vi "Create Tree.vi"(8 "Error In":errorcluster, 10 "Graves":T1[](array[typedef]), 11 "TreeControl In":refnum<vi>) -> (0 "Error Out":errorcluster, 3 "TreeControl Out":refnum<vi>)   [LabVIEW 2017, in "Graveyard.lvlib"]
uses:
  Graveyard.lvlib
  VI Bookmark.ctl
  VI Information.ctl
  Application Information.ctl
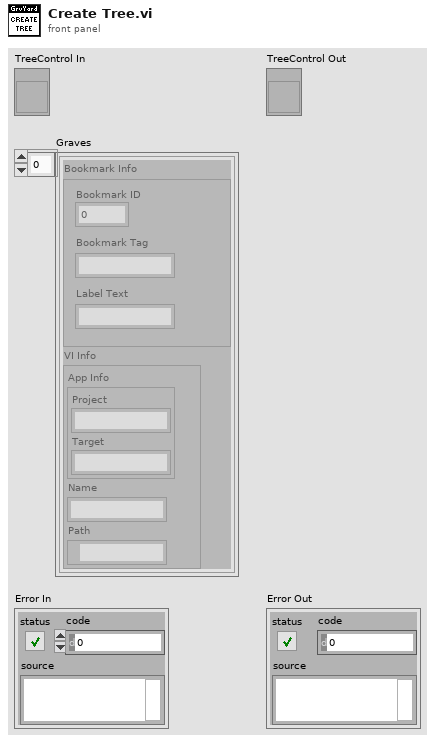
[diagram p1: front panel]
types:
  T1 = typedef "Graveyard.lvlib/VI Bookmark.ctl" = cluster{"Bookmark Info":cluster{"Bookmark ID":u32, "Bookmark Tag":string, "Label Text":string}, "VI Info":T2}
  T2 = typedef "Graveyard.lvlib/VI Information.ctl" = cluster{"App Info":T3, "Name":string, "Path":path}
  T3 = typedef "Graveyard.lvlib/Application Information.ctl" = cluster{"Project":string, "Target":string}
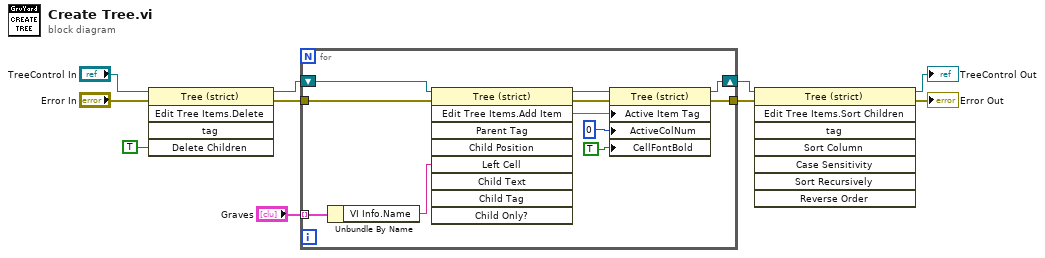
[diagram p0: block diagram]
diagram:
  n1 = invoke class="Tree (strict)" method="Edit Tree Items.Delete"(reference="TreeControl In", error in="Error In", "Delete Children"=TRUE ("Delete Children?")) -> (reference out=w5:refnum<vi>, error out=w7:errorcluster)  [unwired: 2 in, 3 out]
  n2 = for {
    shift-right: [w17] -> w6
    shift-left: w5 -> [w20]
    tunnel: w7 -> [w21]
    tunnel: [w15] -> w9
    tunnel: "Graves" -> [w11] mode=indexing
    n3 = Unbundle By Name(w11) -> ("VI Info.Name"=w18:string)
    n4 = invoke class="Tree (strict)" method="Edit Tree Items.Add Item"(reference=w20, error in=w21, "Left Cell"=w18) -> (reference out=w19:refnum<vi>, error out=w16:errorcluster, "Edit Tree Items:Add Item"=w12:string)  [unwired: 6 in, 6 out]
    n5 = property class="Tree (strict)"(reference=w19, error in=w16, "Active Item Tag"=w12, "ActiveColNum"=0 ("Active Cell:Active Column Number"), "CellFontBold"=TRUE ("Active Cell:Cell Font:Bold")) -> (reference out=w17:refnum<vi>, error out=w15:errorcluster)
  }
  n6 = invoke class="Tree (strict)" method="Edit Tree Items.Sort Children"(reference=w6, error in=w9) -> (reference out=→"TreeControl Out":refnum<vi>, error out=→"Error Out":errorcluster)  [unwired: 6 in, 6 out]
